vi "Update Cooker Duration.vi"(8 "error in (no error)":errorcluster, 10 "Duration (s)":dbl format="%.2f s", 11 "Cooker Actor in":refnum<class "Cooker Actor.lvclass">) -> (0 "error out":errorcluster, 3 "Cooker Actor out":refnum<class "Cooker Actor.lvclass">)   [LabVIEW 2024, in "Cooker Actor.lvlib" / "Cooker Actor.lvclass"]
uses:
  Cooker Actor.lvclass
  Cooker Actor.lvclass/Cooker Actor.ctl
  <vilib>/ActorFramework/Actor/Actor.lvclass
  Kitchen Messaging Interface/Kitchen Messaging Interface Messages/Update Timer Msg/Update Timer Msg.lvclass
  C:/Program Files/National Instruments/LabVIEW 2024/vi.lib/ActorFramework/Actor/Actor.lvclass
  C:/Users/burakkorkmaz/Desktop/Leveling/repo/Cooker Actor/Cooker Actor/Cooker Actor.lvclass
  C:/Users/burakkorkmaz/Desktop/Leveling/repo/Cooker Messaging Interface/Cooker Messaging Interface/Cooker Messaging Interface.lvclass
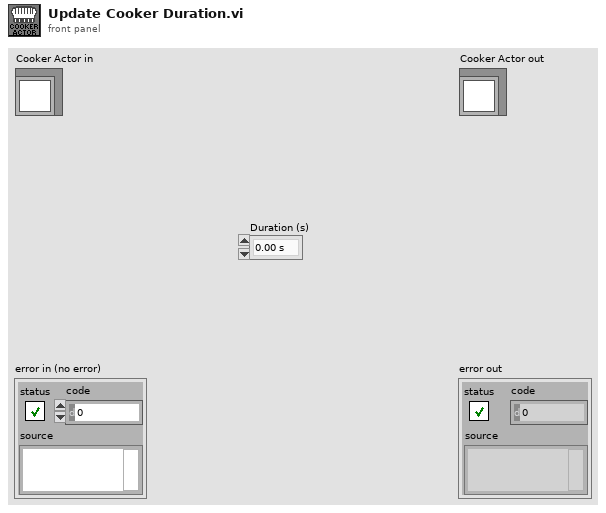
[diagram p1: front panel]
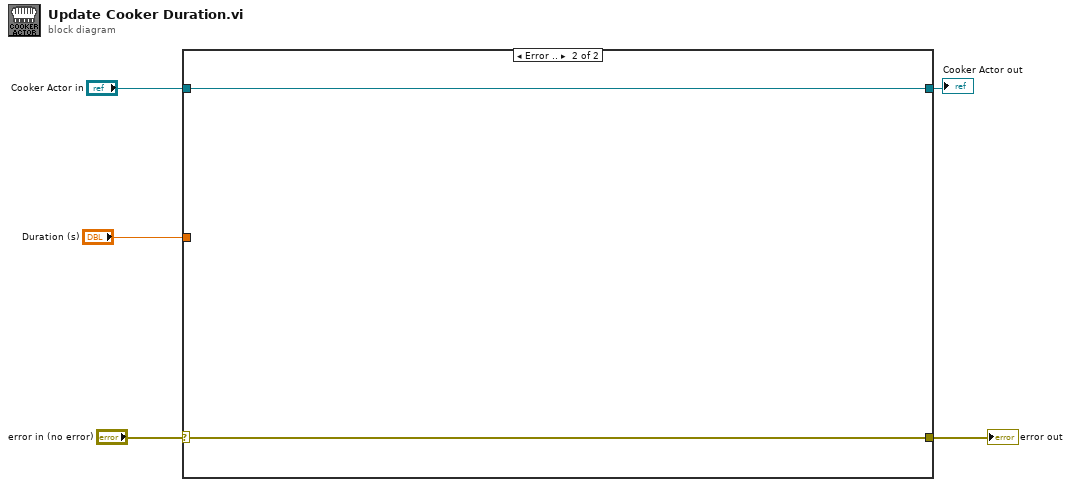
[diagram p0: block diagram]
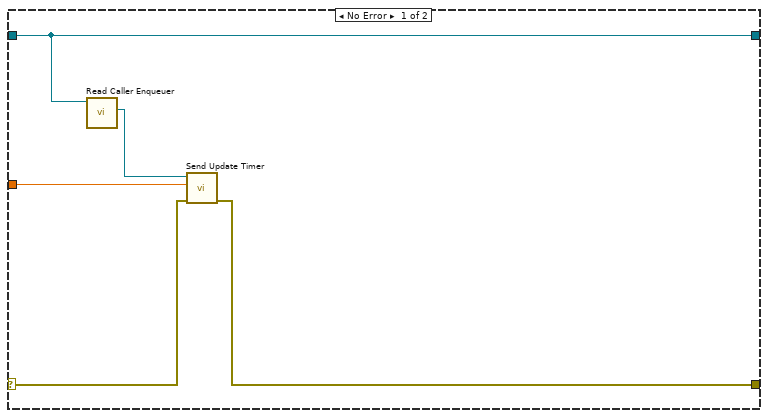
[diagram p2: hidden frame]
diagram:
  n1 = case shown="Error .." "error in (no error)" {
    selector: "error in (no error)" -> [w10 w11]
    tunnel: [w8 w11] -> w4
    tunnel: "Cooker Actor in" -> [w9 w12]
    tunnel: [w9 w12] -> w2
    tunnel: "Duration (s)" -> [w6 _]
    frame No Error {
      n2 = call <vilib>:"Read Caller Enqueuer.vi"("Actor"=w9) -> ("Caller Enqueuer"=w7:refnum<class "Message Enqueuer.lvclass">)  [unwired: 10 in]
      n3 = call "Send Update Timer.vi"("error in (no error)"=w10, "Timer (s)"=w6, "Message Enqueuer"=w7) -> ("error out"=w8:errorcluster)  [unwired: 7 in, 1 out]
    }
    frame Error {
    }
  }
  "error out" <- w4
  "Cooker Actor out" <- w2
